vi "test-DC-Motor-Sim-Test1.vi"() -> (3 "All Passed":bool)   [LabVIEW 2019]
uses:
  <vilib>/Rock Robotics/WPI/ThirdParty/JAS_Junk/TrajLib/Trajectory_Library.lvlib
  <vilib>/Analysis/Matrix/Datatypes/RealMatrix.ctl
  <vilib>/Analysis/Matrix/NI_Matrix.lvlib
  <vilib>/Rock Robotics/WPI/ThirdParty/JAS_Junk/TrajLib/DCMotor_GetNEO.vi
panel:
  out "Zero Speed Passed":bool
  out "Zero Speed":cluster{dbl, "Velocity_RadPerSec":dbl}(graph)
  out "Full Speed Passed":bool
  out "Full Speed":cluster{dbl, "Velocity_RadPerSec":dbl}(graph)
  out "Error":bool
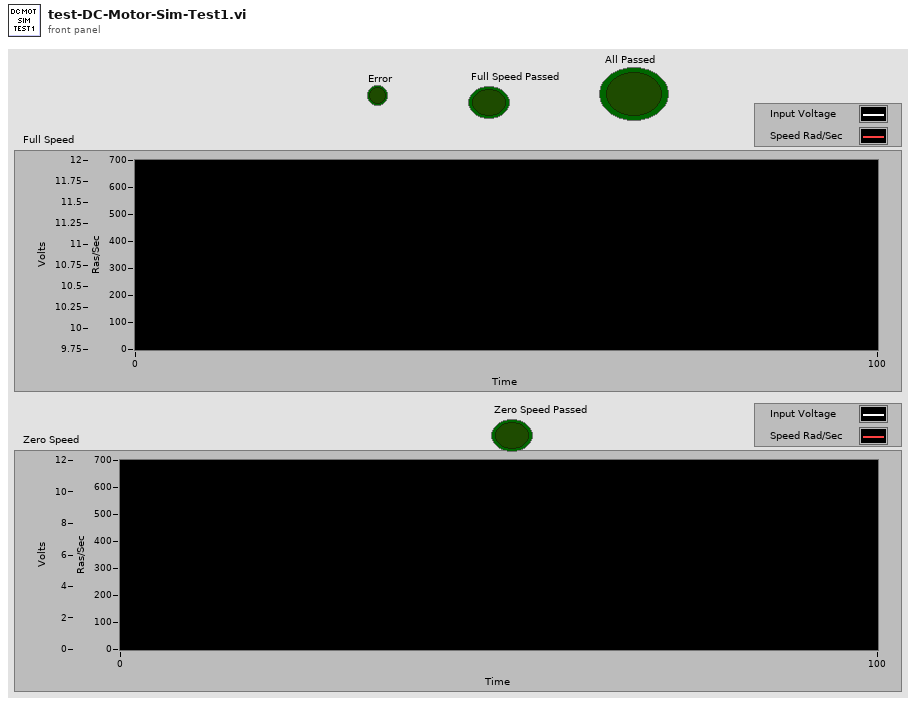
[diagram p1: front panel]
types:
  T1 = typedef "NI_Matrix.lvlib/RealMatrix.ctl" = dbl[][]
  T2 = typedef "Trajectory_Library.lvlib/DCMOTOR.CTL" = cluster{"nominalVoltage_Volts":dbl, "StallTorque_NM":dbl, "StallCurrent_Amps":dbl, "FreeCurrent_Amps":dbl, "FreeSpeed_RadPerSec":dbl, "R_Ohms":dbl, "KvINV_RadPerSecPerVolt":dbl, "Kt_NMPerAmp":dbl, "L_H":dbl, "Jr_KgM2":dbl}
  T3 = typedef "Trajectory_Library.lvlib/DCMOTOR_SIM.ctl" = cluster{"LinearSystemSim":T4, "GearBox":T2, "Gearing":dbl}
  T4 = typedef "Trajectory_Library.lvlib/LINEAR_SYSTEM_SIM.ctl" = cluster{"m_Plant":T5, "m_X":T1, "m_Y":T1, "m_U":T1, "MeasureStdDev":T1}
  T5 = typedef "Trajectory_Library.lvlib/LINEAR_SYSTEM.ctl" = cluster{"m_A":T1, "m_B":T1, "m_C":T1, "m_D":T1, "States":i32, "Inputs":i32, "Outputs":i32}
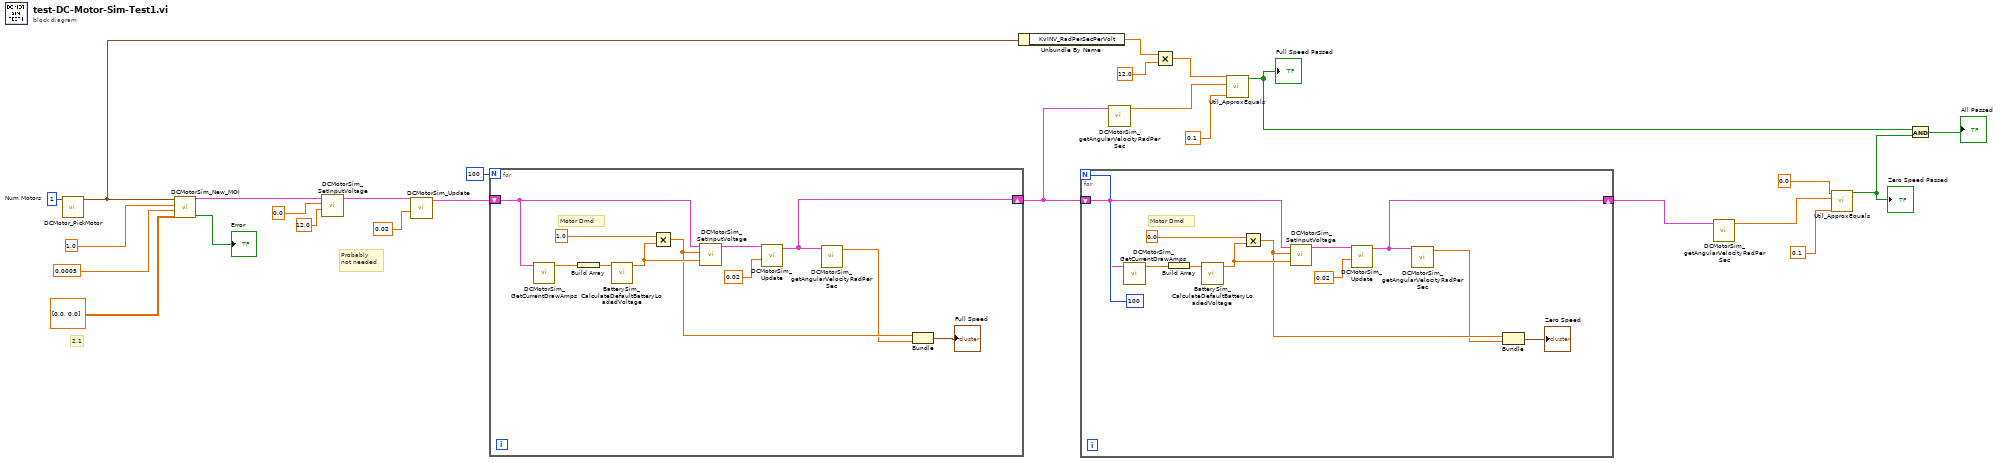
[diagram p0: block diagram]
diagram:
  w27 = 1  # Num Motors
  # "Probably \nnot needed"
  # "2,1"
  n1 = call-poly <vilib>:"DCMotor_PickMotor.vi"("Num Motors"=w27) -> ("DCMOTOR"=w15:T2)  [unwired: 10 in]
  n2 = call <vilib>:"DCMotorSim_New_MOI.vi"("MeasurementStdDev"=T1 [[0.0], [0.0]], "jKgMetersSquared"=0.0005, "Gearing"=1.0, "GearBox"=w15) -> ("Error"=→"Error":bool, "DCMotorSim"=w21:T3)  [unwired: 6 in]
  n3 = call <vilib>:"DCMotorSim_SetInputVoltage.vi"("Battery_Volts"=12.0, "Volts"=0.0, "DCMotorSim"=w21) -> ("out DCMotorSim"=w17:T3)  [unwired: 8 in]
  n4 = call <vilib>:"DCMotorSim_Update.vi"("dT_Seconds"=0.02, "DCMotorSim"=w17) -> ("out DCMotorSim"=w16:T3)  [unwired: 8 in, 1 out]
  n5 = for {
    N: 100 -> [_]
    shift-right: [w28] -> w8
    shift-left: w16 -> [w34]
    # "Motor Dmd"
    n6 = call <vilib>:"DCMotorSim_GetCurrentDrawAmps.vi"("DCMotorSim"=w34) -> ("Current_Amps"=w37:dbl)  [unwired: 10 in]
    n7 = Build Array(w37) -> (w38:dbl[])
    n8 = call <vilib>:"BatterySim_CalculateDefaultBatteryLoadedVoltage.vi"("Currents"=w38) -> ("Voltage"=w36:dbl)  [unwired: 10 in]
    n9 = Multiply(x=1.0, y=w36) -> (x*y=w30:dbl)
    n10 = call <vilib>:"DCMotorSim_SetInputVoltage.vi"("Battery_Volts"=w36, "Volts"=w30, "DCMotorSim"=w34) -> ("out DCMotorSim"=w33:T3)  [unwired: 8 in]
    n11 = call <vilib>:"DCMotorSim_Update.vi"("dT_Seconds"=0.02, "DCMotorSim"=w33) -> ("out DCMotorSim"=w28:T3)  [unwired: 8 in, 1 out]
    n12 = call <vilib>:"DCMotorSim_getAngularVelocityRadPerSec.vi"("DCMotorSim"=w28) -> ("Velocity_RadPerSec"=w29:dbl)  [unwired: 10 in]
    n13 = Bundle(w30, "Velocity_RadPerSec"=w29) -> (→"Full Speed":cluster{dbl, "Velocity_RadPerSec":dbl})  [unwired: 1 in]
  }
  n14 = Unbundle By Name(w15) -> ("KvINV_RadPerSecPerVolt"=w14:dbl)
  n15 = for {
    N: 100 -> [_]
    shift-right: [w39] -> w5
    shift-left: w8 -> [w45]
    # "Motor Dmd"
    n16 = call <vilib>:"DCMotorSim_GetCurrentDrawAmps.vi"("DCMotorSim"=w45) -> ("Current_Amps"=w48:dbl)  [unwired: 10 in]
    n17 = Build Array(w48) -> (w49:dbl[])
    n18 = call <vilib>:"BatterySim_CalculateDefaultBatteryLoadedVoltage.vi"("Currents"=w49) -> ("Voltage"=w47:dbl)  [unwired: 10 in]
    n19 = Multiply(x=0.0, y=w47) -> (x*y=w41:dbl)
    n20 = call <vilib>:"DCMotorSim_SetInputVoltage.vi"("Battery_Volts"=w47, "Volts"=w41, "DCMotorSim"=w45) -> ("out DCMotorSim"=w44:T3)  [unwired: 8 in]
    n21 = call <vilib>:"DCMotorSim_Update.vi"("dT_Seconds"=0.02, "DCMotorSim"=w44) -> ("out DCMotorSim"=w39:T3)  [unwired: 8 in, 1 out]
    n22 = call <vilib>:"DCMotorSim_getAngularVelocityRadPerSec.vi"("DCMotorSim"=w39) -> ("Velocity_RadPerSec"=w40:dbl)  [unwired: 10 in]
    n23 = Bundle(w41, "Velocity_RadPerSec"=w40) -> (→"Zero Speed":cluster{dbl, "Velocity_RadPerSec":dbl})  [unwired: 1 in]
  }
  n24 = call <vilib>:"DCMotorSim_getAngularVelocityRadPerSec.vi"("DCMotorSim"=w8) -> ("Velocity_RadPerSec"=w11:dbl)  [unwired: 10 in]
  n25 = Multiply(x=w14, y=12.0) -> (x*y=w12:dbl)
  n26 = call <vilib>:"Util_ApproxEquals.vi"("Tolerance"=0.1, "Value 2"=w11, "Value 1"=w12) -> ("ApproxEquals"=w2:bool)  [unwired: 8 in]
  "Full Speed Passed" <- w2
  n27 = call <vilib>:"DCMotorSim_getAngularVelocityRadPerSec.vi"("DCMotorSim"=w5) -> ("Velocity_RadPerSec"=w7:dbl)  [unwired: 10 in]
  n28 = call <vilib>:"Util_ApproxEquals.vi"("Tolerance"=0.1, "Value 2"=w7, "Value 1"=0.0 ("y")) -> ("ApproxEquals"=w3:bool)  [unwired: 8 in]
  "Zero Speed Passed" <- w3
  n29 = And(x=w2, y=w3) -> (x .and. y?=→"All Passed":bool)
